vi "VIRBAdll.vi"(8 "error in (no error)":errorcluster, 10 "z":dbl[](array[numeric]), 11 "t":dbl) -> (0 "error out":errorcluster, 3 "ba":dbl)   [LabVIEW 2015]
doc: "subroutine VIRBA (t,x,ba)\n\ncompute second acoustic virial coefficient as a function of temperature\nand composition.\n\nINPUTS:\n t--temperature [K]\n z--composition [array of mol frac]\n\nOUTPUTS:\n ba--second acoustic virial coefficient [L/mol]"
uses:
  REFPROP.dll
panel:
  # "REFPROP-VIRBAdll.vi"
  # "void  VIRBAdll(double *t, double *z, double *ba);"
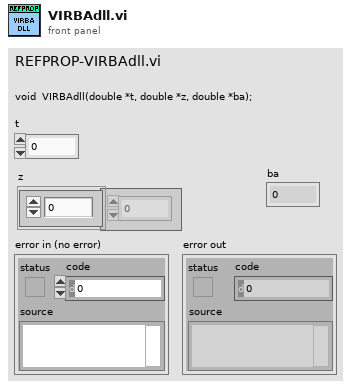
[diagram p1: front panel]
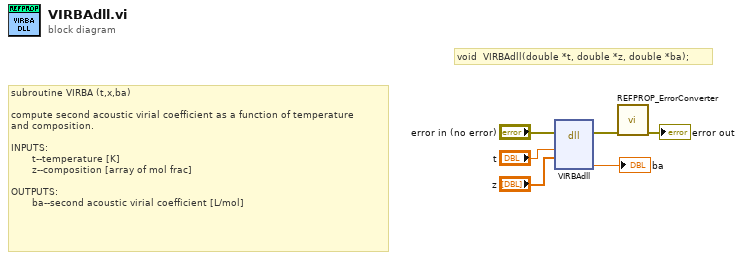
[diagram p0: block diagram]
diagram:
  # "void  VIRBAdll(double *t, double *z, double *ba);"
  # "subroutine VIRBA (t,x,ba)\n\ncompute second acoustic virial coefficient as a function of temperature\nand composition.\n\nINPUTS:\n       t--temperature [K]\n       z--composition [array of mol frac]\n\nOUTPUTS:\n       ba--second acoustic virial coefficient [L/mol]"
  n1 = dll-call lib="C:/Users/lauria/Desktop/REFPROP 10 LabVIEW Wrapper BETA/REFPROP/REFPROP.*" fn="VIRBAdll"(error in="error in (no error)", "t"="t", "z"="z") -> (error out=w3:errorcluster, "ba"=→"ba":dbl)  [unwired: 6 in, 1 out]
  n2 = call "REFPROP_ErrorConverter.vi"("error in (no error)"=w3) -> ("error out"=→"error out":errorcluster)  [unwired: 10 in]
